vi "Get Boolean.vi"(8 "error in (no error)":errorcluster, 11 "ByRef Example in":refnum<class "ByRef Example.lvclass">) -> (0 "error out":errorcluster, 2 "Boolean":bool, 3 "ByRef Example out":refnum<class "ByRef Example.lvclass">)   [LabVIEW 2020, in "ByRef Example.lvclass"]
uses:
  ByRef Example.lvclass
  ByRef Example.lvclass/ByRef Example.ctl
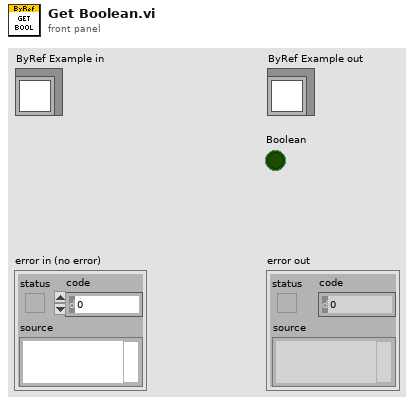
[diagram p1: front panel]
types:
  T1 = typedef "ByRef Example.lvclass/Ref Data.ctl" = cluster{"Boolean":bool, "Numeric":dbl, "String":string}
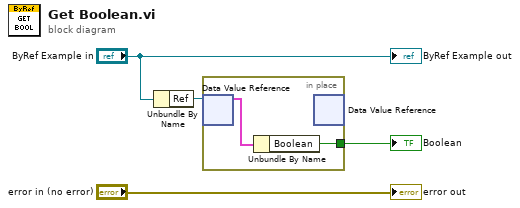
[diagram p0: block diagram]
diagram:
  n1 = Unbundle By Name("ByRef Example in") -> ("Ref"=w2:refnum<data-value>)
  n2 = in-place {
    in-place-border: [w5] -> w1
    n3 = in-place-dvr #1(w2) -> (w6:T1)  [unwired: 1 out]
    n4 = Unbundle By Name(w6) -> ("Boolean"=w5:bool)
    n5 = in-place-dvr #1() -> ()  [unwired: 1 in, 2 out]
  }
  "Boolean" <- w1
  "error out" <- "error in (no error)"
  "ByRef Example out" <- "ByRef Example in"
